vi "GUI_DS-PL1-thermocouple.vi"() -> ()   [LabVIEW 2013]
uses:
  Shared/GUI_Template/GUI_master/tcp_new_data_event.ctl
  Shared/GUI_Template/GUI_master/tcp new data cluster.ctl
panel:
  in  "reading.var 1::1":dbl caption="temperature" min=0.0 max=10000.0
  out "tcp data event":T1
  in  "Refresh Button":bool
  in  "clear":bool
  in  "refresh time (ms)":i32=1000
  out "XY Graph":cluster{timestamp[], dbl[]}(graph)
  in  "stop":bool
  in  "GUIdevice 1":string="PL1-thermocouple"
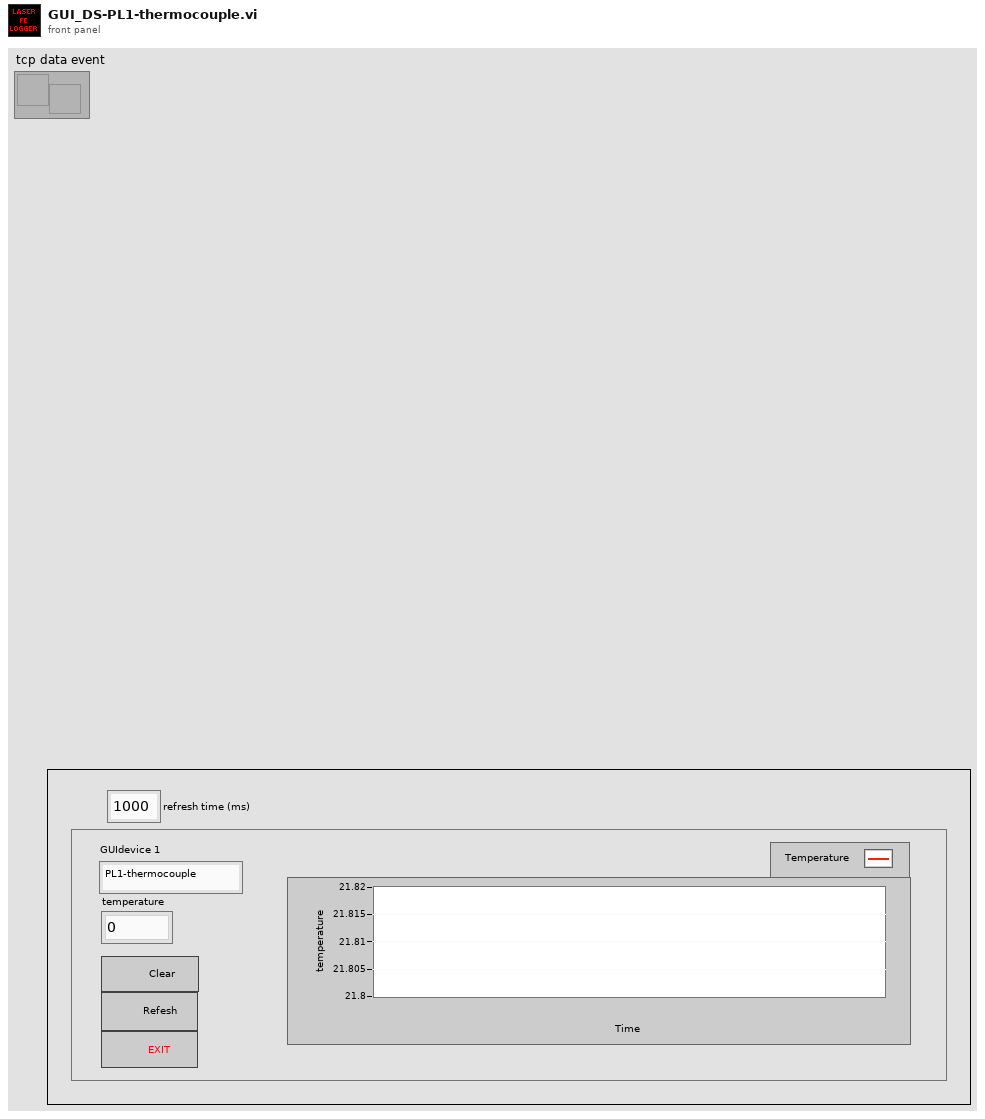
[diagram p1: front panel]
types:
  T1 = typedef "tcp_new_data_event.ctl" = refnum<user-event>
  T2 = enum32{"invalid app kind", "Development System", "Run Time System", "Student Edition", "Embedded LabVIEW", "Evaluation", "Custom"}
  T3 = typedef "tcp new data cluster.ctl" = cluster{"EventEnum":enum16{"new data", "connection status update"}, "Device name":string}
  T4 = enum32{"Invalid", "Standard", "Closed", "Hidden", "Minimized", "Maximized"}
  T5 = cluster{"Core":cluster{"Current VI Reference":refnum<vi>, "Close Panel on Exit?":bool}, "Your Boolean data":bool, "Your string data":string, "SuperGUI":cluster{"STOP queue":refnum<queue>, "SuperGUI ref":refnum<vi>}, "Graph":cluster{"Timestamp":dbl[], "Reading 1":dbl[]}}
  T6 = cluster{"STOP queue":refnum<queue>, "SuperGUI ref":refnum<vi>}
  T7 = cluster{"Current VI Reference":refnum<vi>, "Close Panel on Exit?":bool}
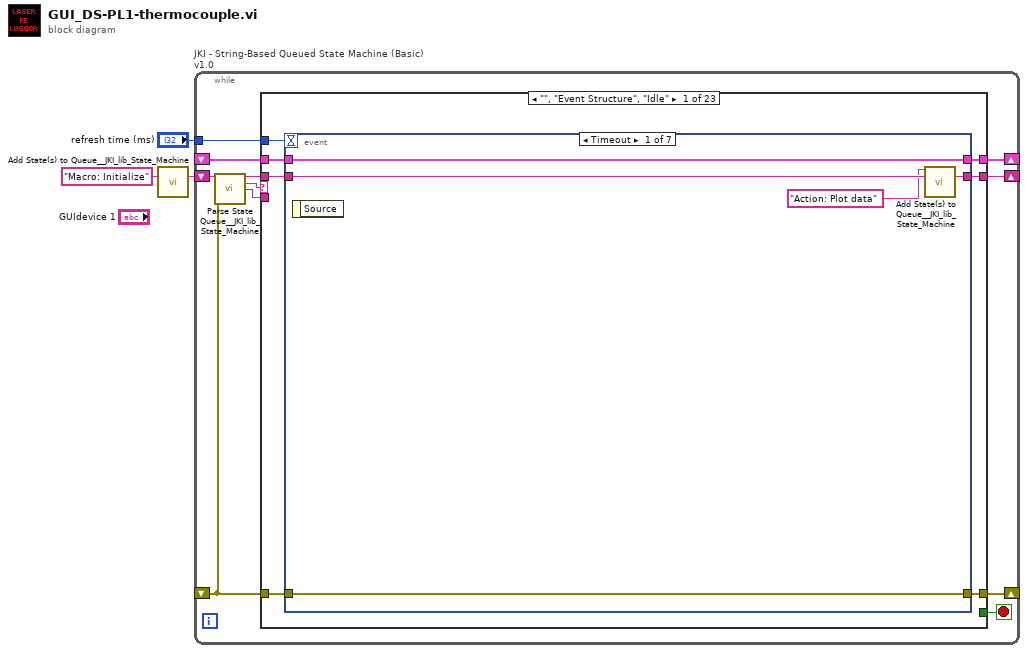
[diagram p0: block diagram]
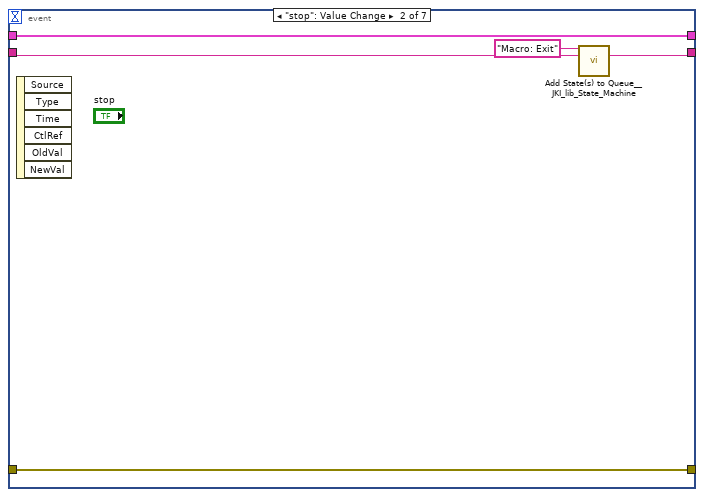
[diagram p2: hidden frame]
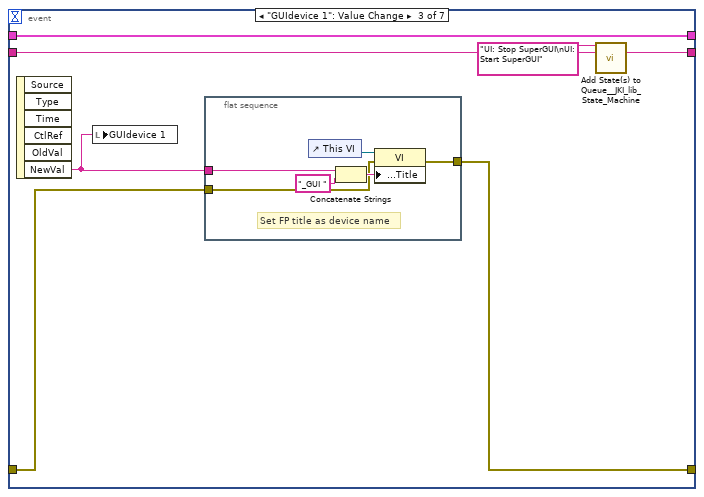
[diagram p3: hidden frame]
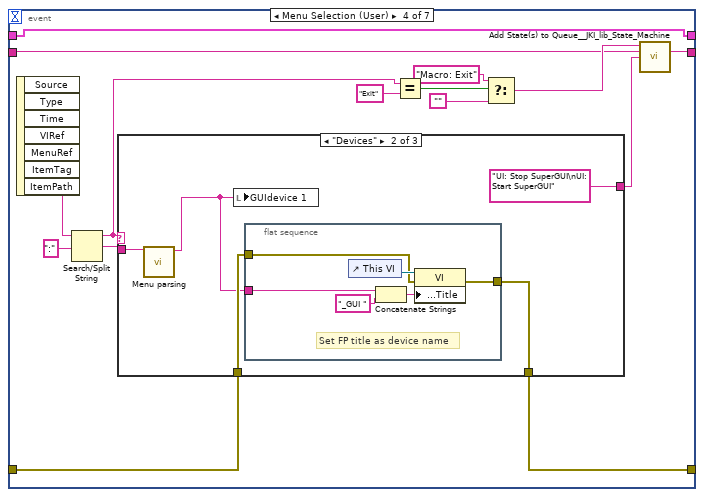
[diagram p4: hidden frame]
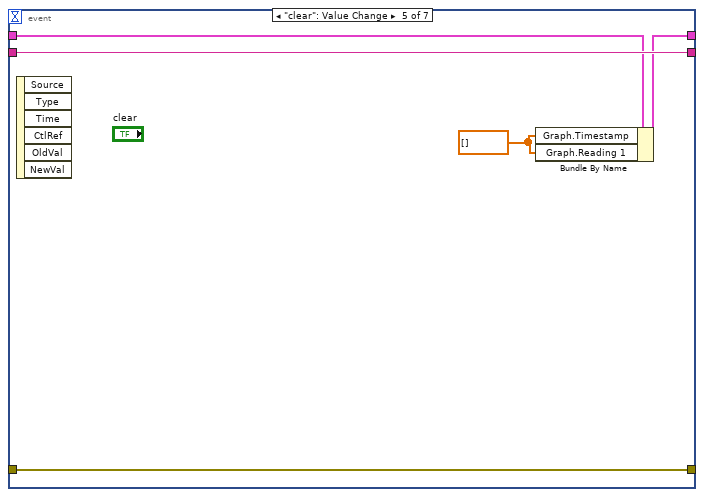
[diagram p7: hidden frame]
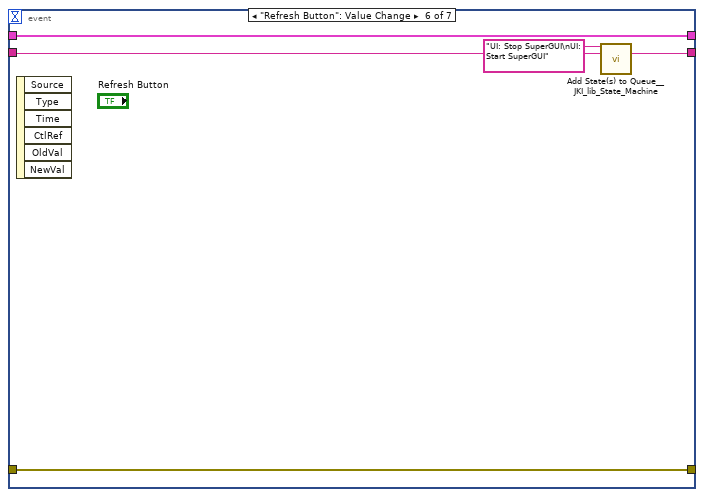
[diagram p8: hidden frame]
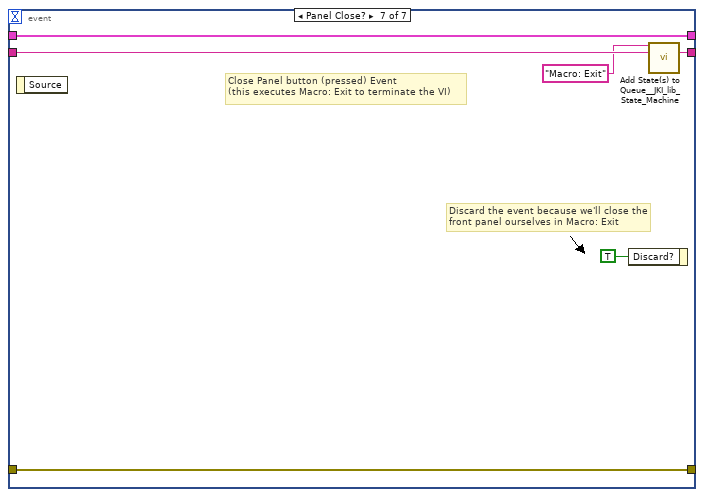
[diagram p9: hidden frame]
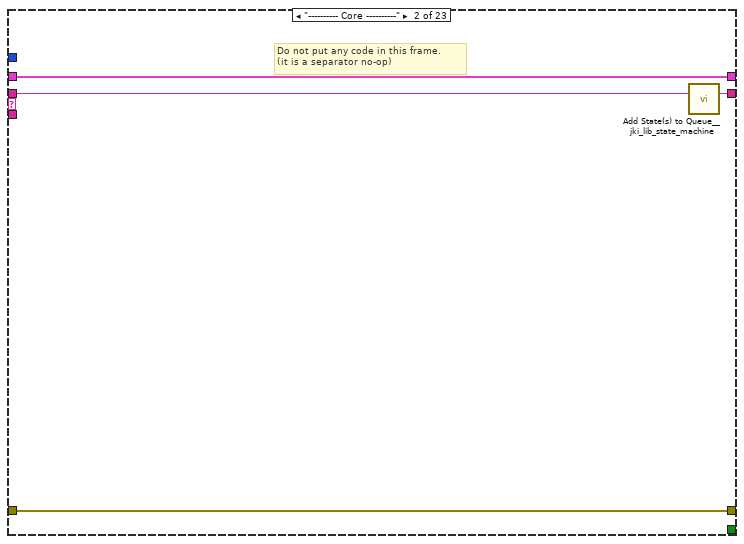
[diagram p10: hidden frame]
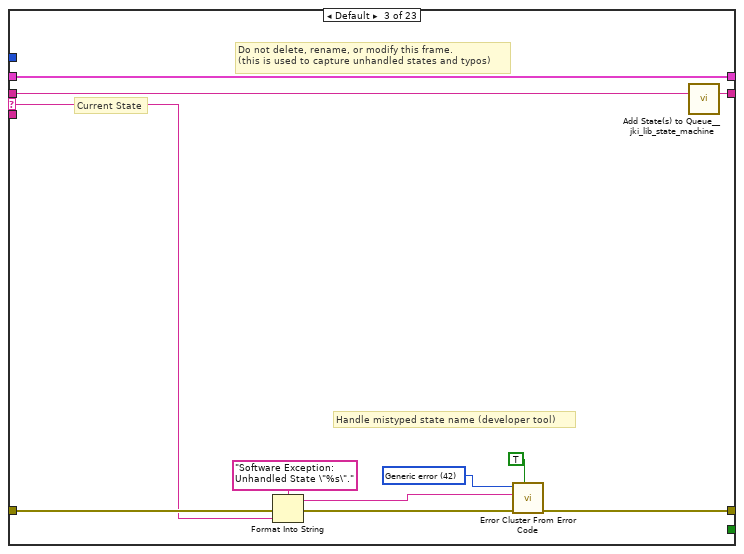
[diagram p11: hidden frame]
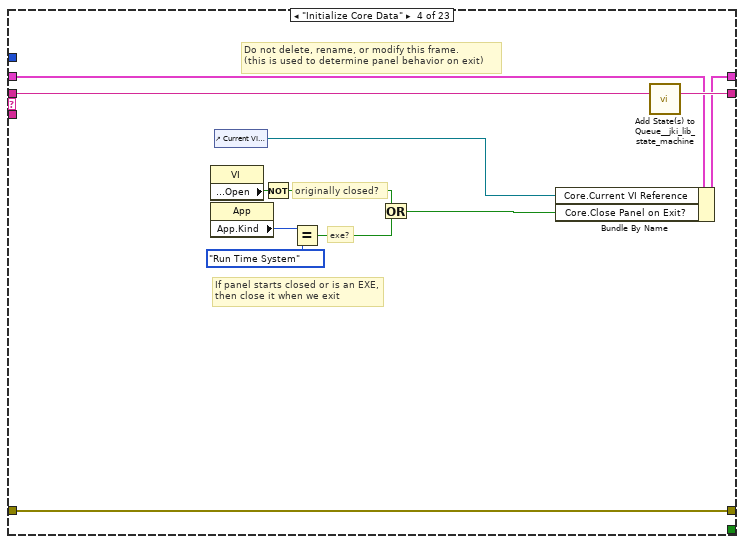
[diagram p12: hidden frame]
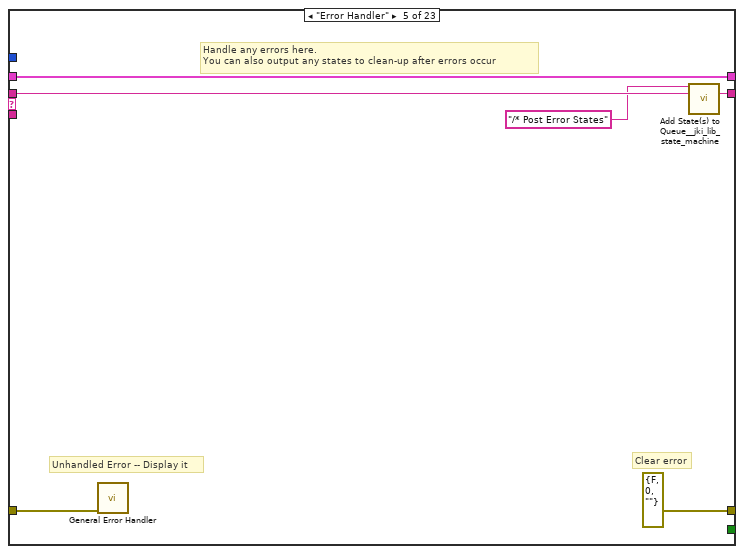
[diagram p13: hidden frame]
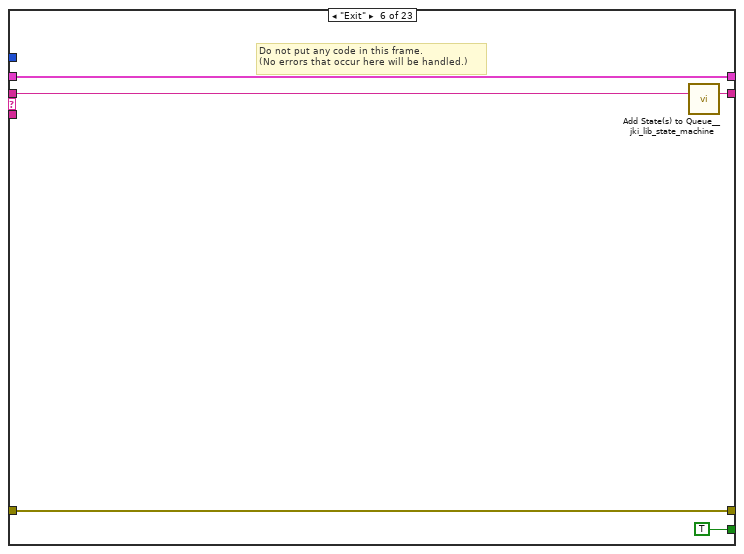
[diagram p14: hidden frame]
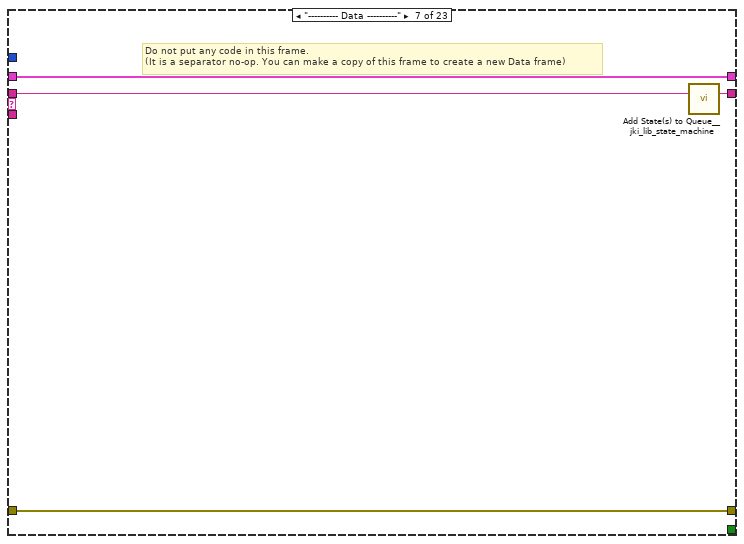
[diagram p15: hidden frame]
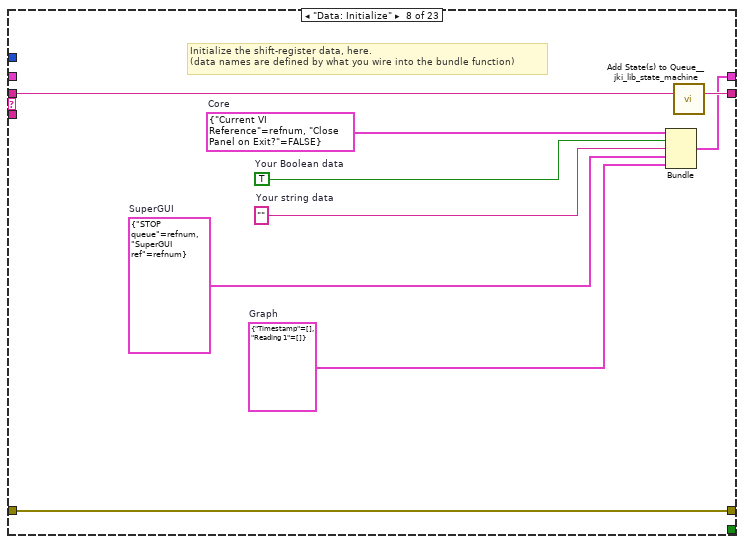
[diagram p16: hidden frame]
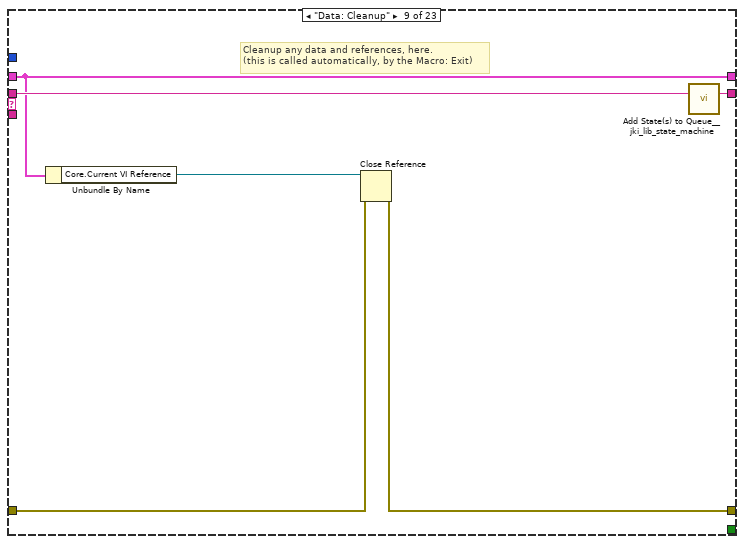
[diagram p17: hidden frame]
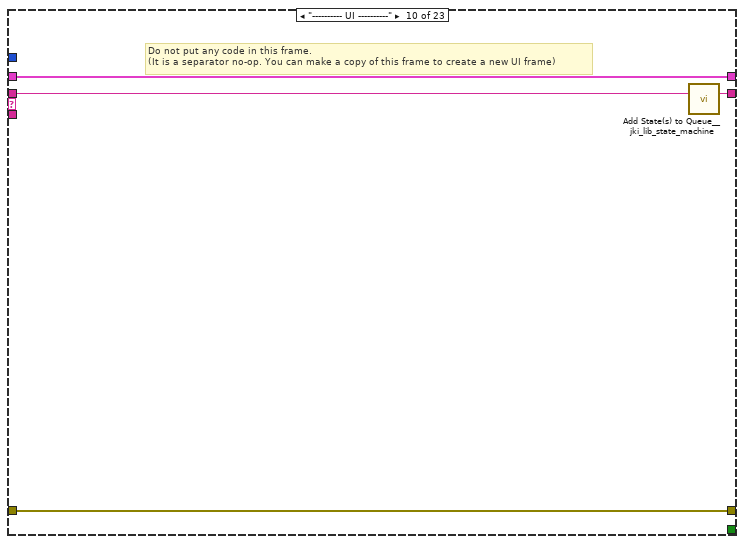
[diagram p18: hidden frame]
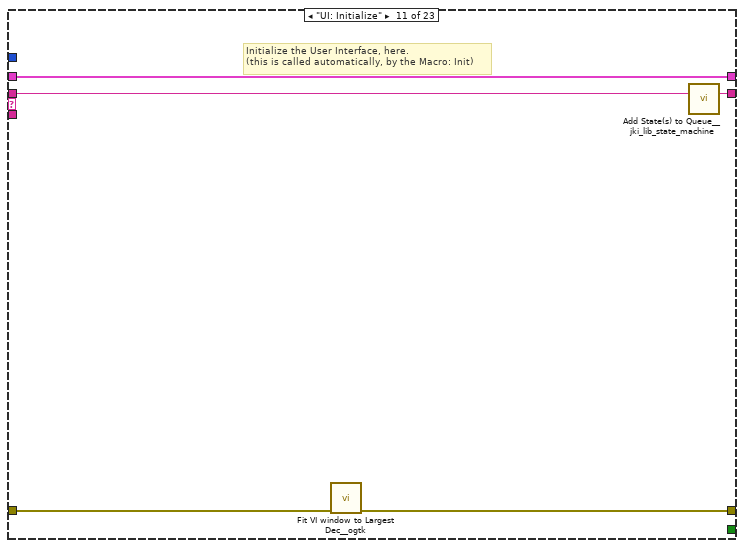
[diagram p19: hidden frame]
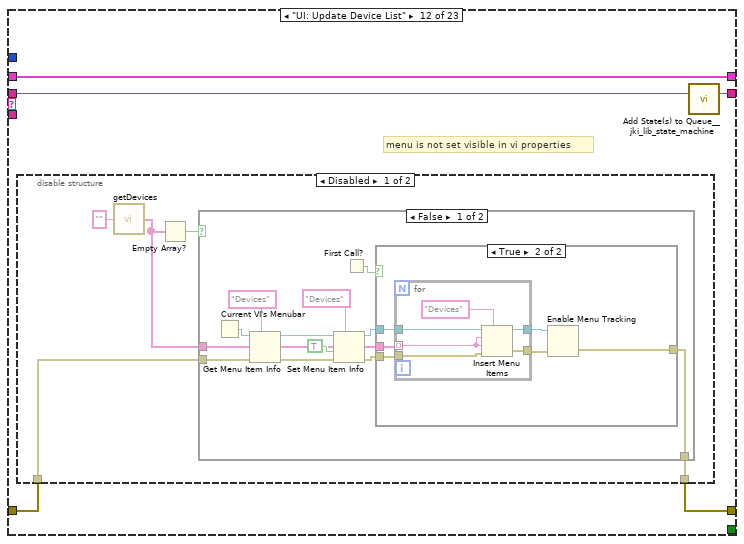
[diagram p20: hidden frame]
diagram:
  n1 = call <vilib>:"Add State(s) to Queue__JKI_lib_State_Machine.vi"("State(s) in (\"\")"="Macro: Initialize") -> ("States Out"=w3:string)  [unwired: 14 in]
  n2 = while "JKI - String-Based Queued State Machine (Basic) v1.0" {
    shift-right: [w7] -> _
    shift-left: _ -> [w6]
    shift-right: [w10] -> _
    shift-left: _ -> [w5]
    shift-right: [w9] -> _
    shift-left: w3 -> [w11]
    tunnel: "refresh time (ms)" -> [w4]
    stop <- w8 stop-if-true
    n3 = call <vilib>:"Parse State Queue__JKI_lib_State_Machine.vi"("State Queue"=w11, "Error In (no error)"=w5) -> ("Remaining States"=w13:string, "Current State"=w14:string, "Arguments"=w12:string)  [unwired: 11 in]
    n4 = case shown="\"\", \"Event Structure\", \"Idle\"" w14 {
      selector: w14 -> [_ _ w93 _ _ _ _ _ _ _ _ _ _ _ _ _ _ _ _ _ _ _ _]
      tunnel: w13 -> [w21 w92 w97 w115 w121 w126 w130 w139 w145 w149 w154 w159 w197 w231 w239 w245 w256 w282 w287 w297 w301 w318 w337]
      tunnel: w12 -> [_ _ _ _ _ _ _ _ _ _ _ _ _ _ _ w240 w250 _ _ _ _ _ _]
      tunnel: w6 -> [w19 w89 w95 w106 w118 w124 w127 _ w140 w146 w152 w157 w195 w222 w234 w243 w252 w279 w284 w294 w298 w305 w334]
      tunnel: [w18 w90 w99 w112 errorcluster {"status"=FALSE, "code"=0, "source"=""} ("error out") w123 w128 w136 w141 w147 w150 w155 w192 w215 w232 w241 w253 w280 w285 w295 w299 w316 w335] -> w10
      tunnel: w5 -> [w17 w90 w98 w112 w117 w123 w128 w136 w142 w147 w151 w156 w193 w216 w233 w242 w254 w280 w285 w295 w299 w316 w335]
      tunnel: [w20 w91 w96 w114 w120 w125 w129 w138 w144 w148 w153 w158 w196 w230 w238 w244 w255 w281 w286 w296 w300 w317 w336] -> w9
      tunnel: [_ _ _ _ _ TRUE _ _ _ _ _ _ _ _ _ _ _ _ _ _ _ _ _] -> w8
      tunnel: [w16 w89 w95 w113 w118 w124 w127 w137 w140 w146 w152 w157 w195 w221 w234 w243 w252 w279 w284 w294 w298 w304 w334] -> w7
      tunnel: w4 -> [w15 _ _ _ _ _ _ _ _ _ _ _ _ _ _ _ _ _ _ _ _ _ _]
      frame "", "Event Structure", "Idle" {
        n5 = event shown="[0] Timeout" {
          selector: _ -> [_ _ _ _ _ _ _]
          dyn-events: _ -> [_ _ _ _ _ _ _]
          timeout: w15 -> [_ _ _ _ _ _ _]
          tunnel: w21 -> [w26 w29 w35 w53 w77 w80 w88]
          tunnel: [w25 w28 w34 w52 w77 w79 w87] -> w20
          tunnel: w19 -> [w23 w31 w38 w59 w75 w82 w85]
          tunnel: [w24 w30 w36 w46 w76 w81 w86] -> w18
          tunnel: w17 -> [w24 w30 w37 w47 w76 w81 w86]
          tunnel: [w23 w31 w38 w59 w74 w82 w85] -> w16
          event Timeout {
            n6 = event-data() -> ()  [unwired: 1 in, 1 out]
            n7 = call <vilib>:"Add State(s) to Queue__JKI_lib_State_Machine.vi"("State(s) in Front (\"\")"="Action: Plot data", "State(s) in (\"\")"=w26) -> ("States Out"=w25:string)  [unwired: 13 in]
          }
          event "stop": Value Change {
            n8 = event-data() -> ()  [unwired: 1 in, 6 out]
            n9 = call <vilib>:"Add State(s) to Queue__JKI_lib_State_Machine.vi"("State(s) in Front (\"\")"="Macro: Exit", "State(s) in (\"\")"=w29) -> ("States Out"=w28:string)  [unwired: 13 in]
          }
          event "GUIdevice 1": Value Change {
            n10 = event-data() -> ("NewVal"=w32:string)  [unwired: 1 in, 5 out]
            n11 = local write "GUIdevice 1"(w32) -> ()
            n12 = flat-sequence {
              tunnel: [w41] -> w36
              tunnel: w37 -> [w40]
              tunnel: w32 -> [w39]
              frame #0 {
                # "Set FP title as device name"
                n13 = control-ref of="This VI"() -> (w44:refnum<vi>)
                n14 = Concatenate Strings(w39, "_GUI ") -> (w43:string)
                n15 = property class="VI"(reference=w44, error in=w40, "Front Panel.Title"=w43) -> (error out=w41:errorcluster)  [unwired: 1 out]
              }
            }
            n16 = call <vilib>:"Add State(s) to Queue__JKI_lib_State_Machine.vi"("State(s) in Front (\"\")"="UI: Stop SuperGUI\nUI: Start SuperGUI", "State(s) in (\"\")"=w35) -> ("States Out"=w34:string)  [unwired: 13 in]
          }
          event Menu Selection (User) {
            n17 = event-data() -> ("ItemPath"=w49:string)  [unwired: 1 in, 6 out]
            n18 = Search/Split String(string=w49, search string/char (-)=":") -> (substring before match=w45:string, match + rest of string=w48:string)  [unwired: 1 in, 1 out]
            n19 = case shown="\"Devices\"" w45 {
              tunnel: w48 -> [_ w65 _]
              tunnel: w47 -> [w60 w64 w72]
              tunnel: [w60 w63 w72] -> w46
              tunnel: [_ "UI: Stop SuperGUI\nUI: Start SuperGUI" _] -> w51
              frame "", Default {
              }
              frame "Devices" {
                n20 = call "Menu parsing.vi"("ItemPath"=w65) -> ("ItemPath"=w61:string)  [unwired: 9 in, 1 out]
                n21 = local write "GUIdevice 1"(w61) -> ()
                n22 = flat-sequence {
                  tunnel: [w68] -> w63
                  tunnel: w64 -> [w67]
                  tunnel: w61 -> [w66]
                  frame #0 {
                    # "Set FP title as device name"
                    n23 = control-ref of="This VI"() -> (w71:refnum<vi>)
                    n24 = Concatenate Strings(w66, "_GUI ") -> (w70:string)
                    n25 = property class="VI"(reference=w71, error in=w67, "Front Panel.Title"=w70) -> (error out=w68:errorcluster)  [unwired: 1 out]
                  }
                }
              }
              frame "Exit" {
              }
            }
            n26 = Equal?(x=w45, y="Exit") -> (x = y?=w57:bool)
            n27 = Select(t="Macro: Exit", s=w57, f="") -> (s? t:f=w54:string)
            n28 = call <vilib>:"Add State(s) to Queue__JKI_lib_State_Machine.vi"("State(s) in Front (\"\")"=w54, "State(s) in (\"\")"=w53, "State(s) at Back (\"\")"=w51) -> ("States Out"=w52:string)  [unwired: 12 in]
          }
          event "clear": Value Change {
            w73 = dbl[] [] ("Array")
            n29 = event-data() -> ()  [unwired: 1 in, 6 out]
            n30 = Bundle By Name(cluster=w75, "Graph.Timestamp"=w73, "Graph.Reading 1"=w73) -> (w74:T5)
          }
          event "Refresh Button": Value Change {
            n31 = event-data() -> ()  [unwired: 1 in, 6 out]
            n32 = call <vilib>:"Add State(s) to Queue__JKI_lib_State_Machine.vi"("State(s) in Front (\"\")"="UI: Stop SuperGUI\nUI: Start SuperGUI", "State(s) in (\"\")"=w80) -> ("States Out"=w79:string)  [unwired: 13 in]
          }
          event Panel Close? {
            # "Discard the event because we'll close the front panel ourselves in Macro: Exit"
            # "Close Panel button (pressed) Event\n(this executes Macro: Exit to terminate the VI)"
            n33 = event-data() -> ()  [unwired: 1 in, 1 out]
            n34 = event-data("Discard?"=TRUE) -> ()  [unwired: 1 in, 1 out]
            n35 = call <vilib>:"Add State(s) to Queue__JKI_lib_State_Machine.vi"("State(s) in Front (\"\")"="Macro: Exit", "State(s) in (\"\")"=w88) -> ("States Out"=w87:string)  [unwired: 13 in]
          }
        }
      }
      frame "---------- Core ----------" {
        # "Do not put any code in this frame.\n(it is a separator no-op)"
        n36 = call <vilib>:"Add State(s) to Queue__jki_lib_state_machine.vi"("State(s) in (\"\")"=w92) -> ("States Out"=w91:string)  [unwired: 14 in]
      }
      frame Default {
        w102 = 42 items=["No error", "Argument error", "Memory is full", "Out of zone", "End of file", "File already open", "Generic file I/O error", "File not found", "File permission error", "Disk is full", "Duplicate path", "Too many files open", "System feature not enabled", "Resource file not found", "Cannot add resource", "Resource not found", "Image not found", "Image memory error", "Pen does not exist", "Config type invalid", "Config token not found", "Config parse error", "Config memory error", "Bad external code format", "Bad external code offset", "External code not present", "Null window", "Destroy window error", "Null menu", "Print aborted", "Bad print record", "Print driver error", "Windows error during printing", "Memory error during printing", "Print dialog error", "Generic print error", "Invalid device refnum", "Device not found", "Device parameter error", "Device unit error", "Cannot open device", "Device call aborted", "Generic error", "Cancelled by user", "Object ID too low", "Object ID too high", "Object not in heap", "Unknown heap", "Unknown object (invalid DefProc)", "Unknown object (DefProc not in table)", "Message out of range", "Invalid (null) method", "Unknown message", "Manager call not supported", "Bad address", "Network operation in progress", "Network operation timed out", "Connection is busy", "Network attribute not supported", "Network error", "Address in use", "System out of memory", "Connection aborted", "Connection refused", "Not connected", "Already connected", "Connection closed", "Initialization error (interapplication manager)", "Bad occurrence", "Wait on unbound occurrence handler", "Occurrence queue overflow", "Datalog type conflict", "Unused", "Unrecognized type (interapplication manager)", "Memory corrupt", "Failed to make temporary DLL", "Old CIN version", "Drag socket not found", "Failed to load drop-object", "Failed to register OLE object", "Failed to release OLE object", "Format specifier type mismatch", "Unknown format specifier", "Too few format specifiers", "Too many format specifiers", "Scan failed", "Newer CIN version", "Error converting to variant", "Runtime menu error", "Password tampered", "Variant attribute not found", "Incompatible variant data type", "Event data is not available", "Event Store is not present", "Occurrence is not found", "Event Queue is not created", "Event info is not available", "Refnum passed is NULL", "Error retrieving Class GUID", "Error retrieving CoClass GUID", "Error retrieving TypeLib GUID.", "Bad built application magic bytes.", "Specific driver is different from the specific driver associated with the Logical Name.", "There is no session opened to the class driver.", "Max Error", "MAX - Error with config objects", "MAX - Error loading configuration", "MAX - Group not supported"]
        # "Current State"
        # "Do not delete, rename, or modify this frame.\n(this is used to capture unhandled states and typos)"
        # "Handle mistyped state name (developer tool)"
        n37 = Format Into String(format string="Software Exception: Unhandled State \"%s\"." ("message"), error in=w98, w93) -> (resulting string=w101:string, error out=w100:errorcluster)  [unwired: 1 in]
        n38 = call <vilib>:"Error Cluster From Error Code.vi"("show call chain? (False)"=TRUE, "error in (no error)"=w100, "error message (\"\")"=w101, "error code (0)"=w102) -> ("error out"=w99:errorcluster)  [unwired: 5 in]
        n39 = call <vilib>:"Add State(s) to Queue__jki_lib_state_machine.vi"("State(s) in (\"\")"=w97) -> ("States Out"=w96:string)  [unwired: 14 in]
      }
      frame "Initialize Core Data" {
        # "Do not delete, rename, or modify this frame.\n(this is used to determine panel behavior on exit)"
        # "originally closed?"
        # "exe?"
        # "If panel starts closed or is an EXE, then close it when we exit"
        n40 = property class="VI"() -> ("Front Panel.Open"=w111:bool)  [unwired: 2 in, 2 out]
        n41 = property class="App"() -> ("App.Kind"=w110:T2)  [unwired: 2 in, 2 out]
        n42 = control-ref of="Current VI Reference"() -> (w104:refnum<vi>)
        n43 = Not(x=w111) -> (.not. x?=w108:bool)
        n44 = Equal?(x=w110, y=T2."Run Time System" ("Application:Kind")) -> (x = y?=w107:bool)
        n45 = Or(x=w108, y=w107) -> (x .or. y?=w105:bool)
        n46 = Bundle By Name(cluster=w106, "Core.Current VI Reference"=w104, "Core.Close Panel on Exit?"=w105) -> (w113:T5)
        n47 = call <vilib>:"Add State(s) to Queue__jki_lib_state_machine.vi"("State(s) in (\"\")"=w115) -> ("States Out"=w114:string)  [unwired: 14 in]
      }
      frame "Error Handler" {
        # "Unhandled Error -- Display it"
        # "Handle any errors here.\nYou can also output any states to clean-up after errors occur"
        # "Clear error"
        n48 = call <vilib>:"General Error Handler.vi"("error in (no error)"=w117) -> ()  [unwired: 10 in, 5 out]
        n49 = call <vilib>:"Add State(s) to Queue__jki_lib_state_machine.vi"("State(s) in Front (\"\")"="/* Post Error States", "State(s) in (\"\")"=w121) -> ("States Out"=w120:string)  [unwired: 13 in]
      }
      frame "Exit" {
        # "Do not put any code in this frame.\n(No errors that occur here will be handled.)"
        n50 = call <vilib>:"Add State(s) to Queue__jki_lib_state_machine.vi"("State(s) in (\"\")"=w126) -> ("States Out"=w125:string)  [unwired: 14 in]
      }
      frame "---------- Data ----------" {
        # "Do not put any code in this frame.\n(It is a separator no-op. You can make a copy of this frame to create a new Data frame)"
        n51 = call <vilib>:"Add State(s) to Queue__jki_lib_state_machine.vi"("State(s) in (\"\")"=w130) -> ("States Out"=w129:string)  [unwired: 14 in]
      }
      frame "Data: Initialize" {
        w131 = cluster{"Timestamp":dbl[], "Reading 1":dbl[]} {"Timestamp"=[], "Reading 1"=[]}  # Graph
        w132 = T6 {"STOP queue"=refnum, "SuperGUI ref"=refnum}  # SuperGUI
        w133 = T7 {"Current VI Reference"=refnum, "Close Panel on Exit?"=FALSE}  # Core
        w135 = TRUE  # Your Boolean data
        w134 = ""  # Your string data
        # "Initialize the shift-register data, here.\n(data names are defined by what you wire into the bundle function)"
        n52 = Bundle("Core"=w133, "Your Boolean data"=w135, "Your string data"=w134, "SuperGUI"=w132, "Graph"=w131) -> (w137:T5)  [unwired: 1 in]
        n53 = call <vilib>:"Add State(s) to Queue__jki_lib_state_machine.vi"("State(s) in (\"\")"=w139) -> ("States Out"=w138:string)  [unwired: 14 in]
      }
      frame "Data: Cleanup" {
        # "Cleanup any data and references, here.\n(this is called automatically, by the Macro: Exit)"
        n54 = Unbundle By Name(w140) -> ("Core.Current VI Reference"=w143:refnum<vi>)
        n55 = Close Reference(reference=w143, error in (no error)=w142) -> (error out=w141:errorcluster)
        n56 = call <vilib>:"Add State(s) to Queue__jki_lib_state_machine.vi"("State(s) in (\"\")"=w145) -> ("States Out"=w144:string)  [unwired: 14 in]
      }
      frame "---------- UI ----------" {
        # "Do not put any code in this frame.\n(It is a separator no-op. You can make a copy of this frame to create a new UI frame)"
        n57 = call <vilib>:"Add State(s) to Queue__jki_lib_state_machine.vi"("State(s) in (\"\")"=w149) -> ("States Out"=w148:string)  [unwired: 14 in]
      }
      frame "UI: Initialize" {
        # "Initialize the User Interface, here.\n(this is called automatically, by the Macro: Init)"
        n58 = call <userlib>:"Fit VI window to Largest Dec__ogtk.vi"("error in (no error)"=w151) -> ("error out"=w150:errorcluster)  [unwired: 5 in, 1 out]
        n59 = call <vilib>:"Add State(s) to Queue__jki_lib_state_machine.vi"("State(s) in (\"\")"=w154) -> ("States Out"=w153:string)  [unwired: 14 in]
      }
      frame "UI: Update Device List" {
        # "menu is not set visible in vi properties"
        n60 = disable-structure shown="Disabled" {
          disable-tunnel: w156 -> [w164 w191]
          disable-tunnel: [w162 w191] -> w155
          frame Disabled {
            n61 = call "getDevices.vi"("Device Class"="") -> ("All Devices"=w160:string[])
            n62 = Empty Array?(array=w160) -> (empty?=w161:bool)
            n63 = case shown="False" w161 {
              tunnel: w164 -> [w167 w190]
              tunnel: [w166 w190] -> w162
              tunnel: w160 -> [w165 _]
              frame False {
                n64 = Current VI's Menubar() -> (w170:refnum<k9>)
                n65 = Get Menu Item Info(7:"Devices" ("item tag"), 8:w167, 11:w170) -> (0:w176:errorcluster, 3:w172:refnum<k9>)  [unwired: 5 out]
                n66 = Set Menu Item Info(7:"Devices" ("item tag"), 8:w176, 9:TRUE ("enabled"), 11:w172) -> (0:w175:errorcluster, 3:w174:refnum<k9>)  [unwired: 3 in]
                n67 = First Call?() -> (First Call?: T/F=w168:bool)
                n68 = case shown="True" w168 {
                  tunnel: w174 -> [_ w182]
                  tunnel: w165 -> [_ w181]
                  tunnel: w175 -> [w177 w179]
                  tunnel: [w177 w178] -> w166
                  frame False {
                  }
                  frame True {
                    n69 = for {
                      tunnel: [w189] -> w183
                      tunnel: w181 -> [w187] mode=indexing
                      tunnel: w182 -> [w186]
                      tunnel: [w185] -> w180
                      tunnel: w179 -> [w184]
                      n70 = Insert Menu Items(5:"Devices" ("menu tag"), 6:w184, 7:w187, 8:w187, 9:w186) -> (0:w185:errorcluster, 3:w189:refnum<k9>)  [unwired: 1 in, 1 out]
                    }
                    n71 = Enable Menu Tracking(2:w180, 4:w183) -> (0:w178:errorcluster)  [unwired: 1 in, 1 out]
                  }
                }
              }
              frame True {
              }
            }
          }
          frame Enabled {
          }
        }
        n72 = call <vilib>:"Add State(s) to Queue__jki_lib_state_machine.vi"("State(s) in (\"\")"=w159) -> ("States Out"=w158:string)  [unwired: 14 in]
      }
      frame "UI: Get Device Name" {
        n73 = First Call?() -> (First Call?: T/F=w194:bool)
        n74 = case shown="True" w194 {
          tunnel: w193 -> [w198 w200]
          tunnel: [w198 w199] -> w192
          frame False {
          }
          frame True {
            n75 = disable-structure "Get Device name from control for vi mode\nand command line arg for exe" shown="RUN_TIME_ENGINE==True" {
              disable-tunnel: w200 -> [_ w202]
              disable-tunnel: [_ w201] -> w199
              frame condition #0 (active) {
              }
              frame condition #1 {
                n76 = control-ref of="This Application"() -> (w210:refnum<vi>)
                n77 = property class="App"(reference=w210) -> ("App.Args"=w209:string[])  [unwired: 1 in, 2 out]
                n78 = Index Array(array=w209, index #1=1 ("index")) -> (element #1=w203:string)  [unwired: 2 in, 2 out]
                n79 = Empty String/Path?(string/path=w203) -> (empty?=w207:bool)
                n80 = control-ref of="This VI"() -> (w206:refnum<vi>)
                n81 = case shown="False" w207 {
                  tunnel: w203 -> [w211 _]
                  frame False {
                    n82 = local write "GUIdevice 1"(w211) -> ()
                  }
                  frame True {
                  }
                }
                n83 = Concatenate Strings(w203, "_GUI ") -> (w205:string)
                n84 = property class="VI"(reference=w206, error in=w202, "Front Panel.Title"=w205) -> (error out=w201:errorcluster)  [unwired: 1 out]
              }
            }
          }
        }
        n85 = call <vilib>:"Add State(s) to Queue__jki_lib_state_machine.vi"("State(s) in (\"\")"=w197) -> ("States Out"=w196:string)  [unwired: 14 in]
      }
      frame "UI: Start SuperGUI" {
        # "create stop queue for supergui and its clones"
        # "x100 abort will be dependent on caller VI\nx80 abort will be independent of caller vi, this will abort vi when labview is closed."
        # "Start SuperGUI asynchronous way"
        n86 = vi-ref "GUI_Master_subvi_reentrant_queues.vi"() -> (w214:refnum<vi>)
        n87 = property class="VI"(reference=w214) -> ("Path"=w213:path)  [unwired: 1 in, 2 out]
        n88 = Create User Event(user event datatype=T3 {"EventEnum"=enum."new data", "Device name"="Device name"} ("New Event"), error in=w216) -> (user event=w217:refnum<user-event>, error out=w223:errorcluster)
        "tcp data event" <- w217
        n89 = control-ref of="This Application"() -> (w220:refnum<vi>)
        n90 = control-ref of="This VI"() -> (w219:refnum<vi>)
        n91 = Open VI Reference(type specifier VI Refnum (for type only)=refnum<vi> refnum, vi path=w213, options=256) -> (vi reference=w229:refnum<vi>, error out=w228:errorcluster)  [unwired: 3 in]
        n92 = register-events(w217) -> ()  [unwired: 2 in, 2 out]
        n93 = call "supergui create stop queue.vi"() -> ("STOP Queue out"=w225:refnum<queue>)  [unwired: 11 in]
        n94 = Current VI's Menubar() -> (w218:refnum<k9>)
        n95 = call-by-ref "Start Asynchronous Call"(reference=w229, error in=w228, "STOP Queue in"=w225, "This Application"=w220, 8:"error in (no error)"=w223, "tcp data event"=w217, "Caller menu reference"=w218, "Caller VI ref"=w219) -> (reference out=w212:refnum<vi>, error out=w215:errorcluster)  [unwired: 5 in, 1 out]
        n96 = Bundle By Name(cluster=w222, "SuperGUI.SuperGUI ref"=w212, "SuperGUI.STOP queue"=w225) -> (w221:T5)
        n97 = call <vilib>:"Add State(s) to Queue__jki_lib_state_machine.vi"("State(s) in (\"\")"=w231) -> ("States Out"=w230:string)  [unwired: 14 in]
      }
      frame "UI: Stop SuperGUI" {
        # "Stop Supergui Clone and wait until it exit properly"
        n98 = Unbundle By Name(w234) -> ("SuperGUI.SuperGUI ref"=w236:refnum<vi>, "SuperGUI.STOP queue"=w235:refnum<queue>)
        n99 = Release Queue(queue=w235, error in (no error)=w233) -> (error out=w237:errorcluster)  [unwired: 1 in, 2 out]
        n100 = call-by-ref "Wait On Asynchronous Call"(reference=w236, error in=w237) -> ("error out"=w232:errorcluster)  [unwired: 11 in, 2 out]
        n101 = call <vilib>:"Add State(s) to Queue__jki_lib_state_machine.vi"("State(s) in (\"\")"=w239) -> ("States Out"=w238:string)  [unwired: 14 in]
      }
      frame "UI: Cursor Set" {
        # "Argument"
        # "Set and Unset Cursor Busy.\n(Usage: \"UI: Cursor Set >> Busy|Idle\")"
        n102 = case shown="\"Idle\", Default" w240 {
          tunnel: w242 -> [w247 w249]
          tunnel: [w246 w248] -> w241
          frame "Idle", Default {
            n103 = call <vilib>:"Unset Busy.vi"("error in (no error)"=w247) -> ("error out"=w246:errorcluster)  [unwired: 10 in]
          }
          frame "Busy" {
            n104 = call <vilib>:"Set Busy.vi"("error in (no error)"=w249) -> ("error out"=w248:errorcluster)  [unwired: 9 in, 1 out]
          }
        }
        n105 = call <vilib>:"Add State(s) to Queue__jki_lib_state_machine.vi"("State(s) in (\"\")"=w245) -> ("States Out"=w244:string)  [unwired: 14 in]
      }
      frame "UI: Front Panel State" {
        # "Argument"
        # "Set Front Panel Open or Closed\n(Usage: \"UI: Front Panel State >> Open|Close\")"
        n106 = Unbundle By Name(w252) -> ("Core.Current VI Reference"=w251:refnum<vi>)
        n107 = case shown="\"Close\"" w250 {
          tunnel: w254 -> [w260 w273]
          tunnel: [w262 w274] -> w253
          tunnel: w251 -> [w261 w271]
          frame "Open", Default {
            n108 = property class="VI"(reference=w261, error in=w260) -> (reference out=w258:refnum<vi>, error out=w259:errorcluster, "Front Panel.Open"=w257:bool)
            n109 = case shown="False" w257 {
              tunnel: [w265 w268] -> w262
              tunnel: w259 -> [w264 w268]
              tunnel: w258 -> [w263 _]
              frame False {
                n110 = invoke class="VI" method="FP.Open"(reference=w263, error in=w264, "Activate"=TRUE, "State"=T4."Standard") -> (error out=w265:errorcluster)  [unwired: 1 in, 4 out]
              }
              frame True {
              }
            }
          }
          frame "Close" {
            n111 = property class="VI"(reference=w271, error in=w273) -> (reference out=w270:refnum<vi>, error out=w272:errorcluster, "Front Panel.Open"=w269:bool)
            n112 = case shown="True" w269 {
              tunnel: [w275 w278] -> w274
              tunnel: w272 -> [w275 w277]
              tunnel: w270 -> [_ w276]
              frame False {
              }
              frame True {
                n113 = invoke class="VI" method="FP.Close"(reference=w276, error in=w277) -> (error out=w278:errorcluster)  [unwired: 1 in, 2 out]
              }
            }
          }
        }
        n114 = call <vilib>:"Add State(s) to Queue__jki_lib_state_machine.vi"("State(s) in (\"\")"=w256) -> ("States Out"=w255:string)  [unwired: 14 in]
      }
      frame "---------- Macro ----------" {
        # "Do not put any code in this frame.\n(It is a separator no-op. You can make a copy of this frame to create a new Macro frame)"
        n115 = call <vilib>:"Add State(s) to Queue__jki_lib_state_machine.vi"("State(s) in (\"\")"=w282) -> ("States Out"=w281:string)  [unwired: 14 in]
      }
      frame "Macro: Initialize" {
        # "Initialization Macro\n(This is called once, when the VI starts)"
        n116 = call <vilib>:"Add State(s) to Queue__jki_lib_state_machine.vi"("State(s) in Front (\"\")"="Data: Initialize\nInitialize Core Data\nUI: Initialize\nUI: Update Device List\nUI: Get Device Name\nUI: Start SuperGUI\nUI: Front Panel State >> Open", "State(s) in (\"\")"=w287) -> ("States Out"=w286:string)  [unwired: 13 in]
      }
      frame "Macro: Exit" {
        # "Exit Macro\n(This is called once, when the VI exits)"
        n117 = Unbundle By Name(w294) -> ("Core.Close Panel on Exit?"=w293:bool)
        n118 = Select(t="UI: Front Panel State >> Close", s=w293, f="") -> (s? t:f=w290:string)
        n119 = call <vilib>:"Add State(s) to Queue__jki_lib_state_machine.vi"("State(s) in (\"\")"=w290, "State(s) at Back (\"\")"="Data: Cleanup\nExit") -> ("States Out"=w288:string)  [unwired: 13 in]
        n120 = call <vilib>:"Add State(s) to Queue__jki_lib_state_machine.vi"("State(s) in Front (\"\")"=w288, "State(s) in (\"\")"=w297) -> ("States Out"=w296:string)  [unwired: 13 in]
      }
      frame "---------- New Category ----------" {
        # "Template Separator\n(You can make a copy of, or modify, this frame)"
        n121 = call <vilib>:"Add State(s) to Queue__jki_lib_state_machine.vi"("State(s) in (\"\")"=w301) -> ("States Out"=w300:string)  [unwired: 14 in]
      }
      frame "Action: Plot data" {
        n122 = Unbundle By Name(w305) -> ("Graph.Timestamp"=w309:dbl[], "Graph.Reading 1"=w308:dbl[])
        n123 = Get Date/Time In Seconds() -> (seconds since 1Jan1904=w313:timestamp)
        n124 = Array Size(array=w309) -> (size(s)=w315:i32)
        n125 = To Double Precision Float(number=w313) -> (double precision float=w311:dbl)
        n126 = Greater?(x=w315, y=14400) -> (0:w312:bool)
        n127 = case shown="True" w312 {
          tunnel: w311 -> [w324 w333]
          tunnel: "reading.var 1::1" -> [w321 w332]
          tunnel: [w323 w326] -> w303
          tunnel: [w322 w325] -> w302
          tunnel: w309 -> [w320 w331]
          tunnel: w308 -> [w319 w330]
          frame False {
            n128 = Build Array (concatenate)(w320, w324) -> (w323:dbl[])
            n129 = Build Array (concatenate)(w319, w321) -> (w322:dbl[])
          }
          frame True {
            w329 = 0
            n130 = Build Array (concatenate)(w331, w333) -> (w328:dbl[])
            n131 = Build Array (concatenate)(w330, w332) -> (w327:dbl[])
            n132 = Delete From Array(array=w328, index=w329) -> (array with subset deleted=w326:dbl[])  [unwired: 1 in, 1 out]
            n133 = Delete From Array(array=w327, index=w329) -> (array with subset deleted=w325:dbl[])  [unwired: 1 in, 1 out]
          }
        }
        n134 = To Time Stamp(1:w303) -> (0:w307:timestamp[])
        n135 = Bundle By Name(cluster=w305, "Graph.Timestamp"=w303, "Graph.Reading 1"=w302) -> (w304:T5)
        n136 = Bundle(w307, w302) -> (→"XY Graph":cluster{timestamp[], dbl[]})  [unwired: 1 in]
        n137 = call <vilib>:"Add State(s) to Queue__jki_lib_state_machine.vi"("State(s) in (\"\")"=w318) -> ("States Out"=w317:string)  [unwired: 14 in]
      }
      frame "New Category: 2" {
        # "Your code here.\n(You can make a copy of, or modify, this frame)"
        n138 = call <vilib>:"Add State(s) to Queue__jki_lib_state_machine.vi"("State(s) in (\"\")"=w337) -> ("States Out"=w336:string)  [unwired: 14 in]
      }
    }
  }
